vi "State Change.vi"(10 "State Transition":refnum<class "State.lvclass">, 11 "State Current":refnum<class "State.lvclass">) -> (0 "error out":errorcluster, 2 "State":refnum<class "State.lvclass">)   [LabVIEW 2021, in "State.lvclass"]
uses:
  State.lvclass
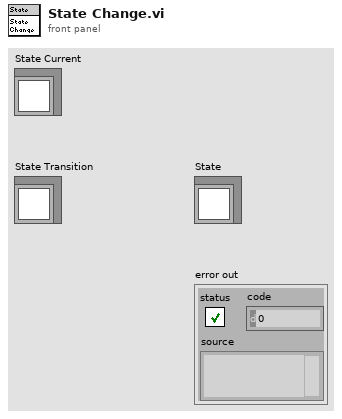
[diagram p1: front panel]
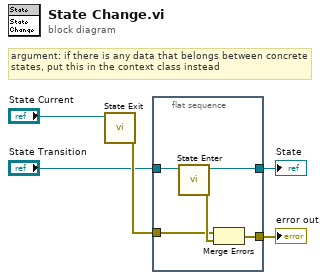
[diagram p0: block diagram]
diagram:
  # "argument: if there is any data that belongs between concrete states, put this in the context class instead"
  n1 = call-dynamic "State Exit.vi"("State in"="State Current") -> ("error out"=w2:errorcluster)  [unwired: 9 in, 1 out]
  n2 = flat-sequence {
    tunnel: [w10] -> w4
    tunnel: [w9] -> w3
    tunnel: w2 -> [w7]
    tunnel: "State Transition" -> [w6]
    frame #0 {
      n3 = call-dynamic "State Enter.vi"("State in"=w6) -> ("error out"=w8:errorcluster, "State out"=w10:refnum<class "State.lvclass">)  [unwired: 9 in]
      n4 = Merge Errors(w7, w8) -> (w9:errorcluster)
    }
  }
  "error out" <- w3
  "State" <- w4
